vi "8-bit video export-Gan AVI info string.vi"(8 "error in (no error)":errorcluster) -> (0 "error out":errorcluster, 3 "Info string":string)   [LabVIEW 2020]
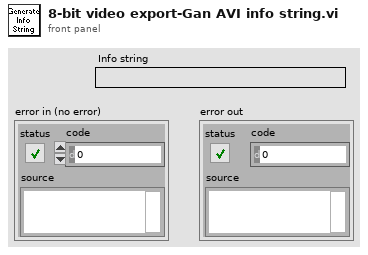
[diagram p1: front panel]
types:
  T1 = typedef "AVI implementation enum.ctl" = enum16{"AVI1", "AVI2"}
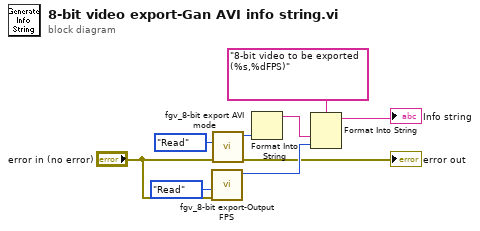
[diagram p0: block diagram]
diagram:
  n1 = call "fgv_8-bit export-Output FPS.vi"("error in (no error)"="error in (no error)", "Function"=enum16{"Intialize", "Write", "Read", "Clear"}."Read") -> ("Frames Per Second"=w9:u32)  [unwired: 8 in, 1 out]
  n2 = call "fgv_8-bit export AVI mode.vi"("error in (no error)"="error in (no error)", "Function"=enum16{"Intialize", "Write", "Read", "Clear"}."Read") -> ("error out"=→"error out":errorcluster, "AVI mode"=w3:T1)  [unwired: 8 in]
  n3 = Format Into String(w3) -> (resulting string=w8:string)  [unwired: 3 in, 1 out]
  n4 = Format Into String(format string="8-bit video to be exported (%s,%dFPS)", w8, w9) -> (resulting string=→"Info string":string)  [unwired: 2 in, 1 out]
